vi "SS2 Live_Image Histogram.vi"() -> ()   [LabVIEW 2019]
uses:
  SS2 Live_Settings List.ctl
  Histograms/Linear Histogram Options.ctl
  Histograms/Histogram Bin Position.ctl
  SS2 DAQ Parameters 3.ctl
  SS2 Gate Definition.ctl
  Calc/Conditional Add 1.llb/Conditional Add 1 [I32].vi
  3eb8dcdc-dfa2-4210-84d8-37bed86b0045.vi/f50f8d4e-175f-4c35-82a4-475d9581d4c4.vi
  3eb8dcdc-dfa2-4210-84d8-37bed86b0045.vi/09f68343-6027-4db5-902e-d62cfc368e59.vi
  3eb8dcdc-dfa2-4210-84d8-37bed86b0045.vi/a7808a9a-c229-4fc4-888b-173237c7e755.vi
  3eb8dcdc-dfa2-4210-84d8-37bed86b0045.vi/34d4bd40-5cc8-4a17-aeb0-05577f0cdd25.vi
  3eb8dcdc-dfa2-4210-84d8-37bed86b0045.vi/9e4b3444-9466-44f3-aaf5-79fcd1be1b69.vi
  3eb8dcdc-dfa2-4210-84d8-37bed86b0045.vi/f50f8d4e-175f-4c35-82a4-475d9581d4c4.vi/53a1494f-7830-4d35-b2a0-1dde755757cb.vi
  GUI/Dialog Window with Option.vi
  <vilib>/Analysis/baseanly.llb/Std Deviation and Variance.vi
  <vilib>/Utility/error.llb/Error Cluster From Error Code.vi
  Variant/Variant to Data/Variant to Data.lvlib
panel:
  out "Image Histogram":cluster{"Axis":dbl[], "Histogram":dbl[]}(graph)
  in  "Stop":bool
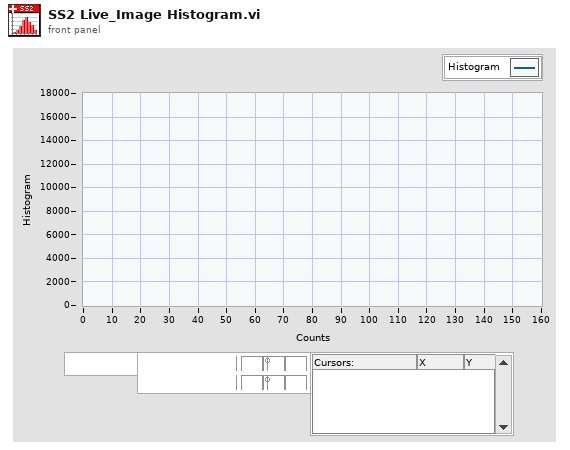
[diagram p1: front panel]
types:
  T1 = typedef "SS2 DAQ Parameters 3.ctl" = cluster{"10 bits":bool, "# Exposure Sequences":u32, "# 1-bit Frame per Gate":u32, "Gate Shift":u32, "# Gates per Set":u32, "# Sets":u32, "Laser Period":dbl[unit], "Sync Period":dbl[unit], "Gate Offset":u32, "Auto-adjust Gate Offset":bool, "Gate Definition":T2}
  T2 = typedef "SS2 Gate Definition.ctl" = cluster{"gs_psincdec_0":u32, "gs_psincdec_1":u32, "gs_psincdec_2":u32, "gs_psincdec_3":u32, "gs_no_shift_adj_1":u32, "gs_no_shift_adj_2":u32, "gs_no_shift_adj_3":u32}
  T3 = typedef "SS2 Live_Settings List.ctl" = enum16{"FPGA:Bitfile Path", "FPGA:Bitfile Version", "FPGA:Auto Reset FPGA", "Acquisition Parameters:SS2 DAQ Parameters", "Acquisition Parameters:Gate Configuration Array", "Acquisition Parameters:Buffer Size (# Gates)", "File Information:File Information", "File Information:# Datasets in Series", "File Information:Scrambled File Flag", "File Information:Delay between Datasets", "Image Parameters:Image ROI Information", "Image Parameters:Image Binning Options", "UI Settings:Histogram Bins Number"}
  T4 = typedef "Linear Histogram Options.ctl" = cluster{"Bin Size":dbl, "Min Value":dbl, "Max Value":dbl, "Filter NaN & Infinite Values":bool, "Frequency Plot":bool, "Align Bins":bool, "Bin Location":T5, "Project Outside Values":bool, "Max Histogram Size":i32}
  T5 = typedef "Histogram Bin Position.ctl" = enum16{"Left", "Center", "Right"}
  T6 = typedef "Array Statistics.ctl" = cluster{"Mean":dbl, "Standard Deviation":dbl, "Max":dbl, "Min":dbl}
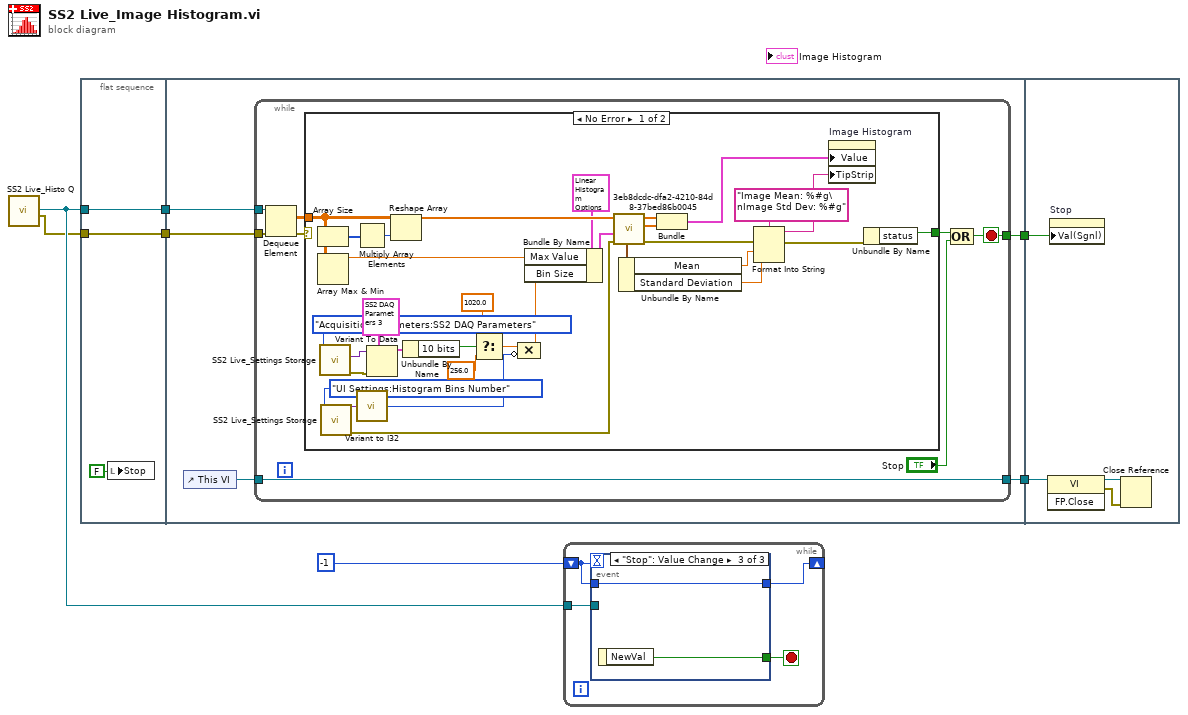
[diagram p0: block diagram]
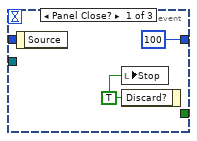
[diagram p2: hidden frame]
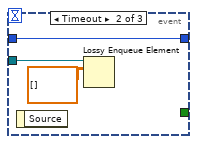
[diagram p3: hidden frame]
diagram:
  n1 = call "SS2 Live_Histo Q.vi"() -> ("error out"=w1:errorcluster, "SS2 Live Histo Q"=w2:refnum<queue>)  [unwired: 6 in]
  n2 = flat-sequence {
    tunnel: [w9] -> w4
    tunnel: w2 -> [w9]
    tunnel: [w8] -> w3
    tunnel: w1 -> [w8]
    tunnel: [w14] -> w7
    tunnel: [w13] -> w6
    tunnel: w4 -> [w12]
    tunnel: w3 -> [w11]
    tunnel: w7 -> [w59]
    tunnel: w6 -> [w58]
    frame #0 {
      n3 = local write "Stop"(FALSE ("Stop")) -> ()
    }
    frame #1 {
      n4 = control-ref of="This VI"() -> (w15:refnum<vi>)
      n5 = while {
        tunnel: w15 -> [w20]
        tunnel: [w20] -> w13
        tunnel: [w18] -> w14
        tunnel: w12 -> [w17]
        tunnel: w11 -> [w16]
        stop <- w18 stop-if-true
        n6 = Dequeue Element(queue=w17, error in (no error)=w16) -> (element=w22:sgl[][], error out=w23:errorcluster)  [unwired: 1 in, 2 out]
        n7 = case shown="No Error" w23 {
          tunnel: w22 -> [w38 _]
          tunnel: [w52 _] -> w21
          frame No Error {
            n8 = Array Size(array=w38) -> (size(s)=w51:i32[])
            n9 = Array Max & Min(array=w38) -> (max value=w36:sgl)  [unwired: 3 out]
            n10 = call "SS2 Live_Settings Storage.vi"("Settings List"=SS2_Live_Settings_List."Acquisition Parameters:SS2 DAQ Parameters") -> ("Error Out"=w33:errorcluster, "Variant Data out"=w32:variant)  [unwired: 9 in]
            n11 = call "SS2 Live_Settings Storage.vi"("Settings List"=SS2_Live_Settings_List."UI Settings:Histogram Bins Number") -> ("Error Out"=w48:errorcluster, "Variant Data out"=w54:variant)  [unwired: 9 in]
            n12 = Multiply Array Elements(1:w51) -> (0:w50:i32)
            n13 = call "Variant to I32.vi"("Variant"=w54) -> ("Value"=w25:i32)  [unwired: 8 in]
            n14 = Variant To Data(error in=w33, type=T1 {"10 bits"=FALSE, "# Exposure Sequences"=0, "# 1-bit Frame per Gate"=255, "Gate Shift"=0, "# Gates per Set"=0, "# Sets"=1, "Laser Period"=0.0, "Sync Period"=0.0, "Gate Offset"=0, "Auto-adjust Gate Offset"=FALSE, "Gate Definition"={"gs_psincdec_0"=0, "gs_psincdec_1"=0, "gs_psincdec_2"=0, "gs_psincdec_3"=0, "gs_no_shift_adj_1"=0, "gs_no_shift_adj_2"=0, "gs_no_shift_adj_3"=0}} ("SS2 DAQ Parameters"), Variant=w32) -> (data=w30:T1)  [unwired: 1 out]
            n15 = Reshape Array(w38, w50) -> (w49:sgl[])
            n16 = Unbundle By Name(w30) -> ("10 bits"=w29:bool)
            n17 = Select(t=1020.0, s=w29, f=256.0) -> (s? t:f=w26:dbl)
            n18 = Compound Arithmetic op=MULTIPLY(w26, invert w25) -> (w24:dbl)
            n19 = Bundle By Name(cluster=T4 {"Bin Size"=nan, "Min Value"=0.0, "Max Value"=inf, "Filter NaN & Infinite Values"=TRUE, "Frequency Plot"=FALSE, "Align Bins"=TRUE, "Bin Location"=enum."Left", "Project Outside Values"=FALSE, "Max Histogram Size"=100000} ("Histogram Options"), "Max Value"=w36, "Bin Size"=w24) -> (w35:T4)
            n20 = call "3eb8dcdc-dfa2-4210-84d8-37bed86b0045.vi"("Error In"=w48, "Histogram Options"=w35, "Array"=w49) -> ("Error Out"=w47:errorcluster, "Array Statistics"=w46:T6, "Histogram"=w42:dbl[], "Axis"=w43:dbl[])  [unwired: 4 in, 1 out]
            n21 = Unbundle By Name(w46) -> ("Mean"=w45:dbl, "Standard Deviation"=w44:dbl)
            n22 = Bundle("Axis"=w43, "Histogram"=w42) -> (w40:cluster{"Axis":dbl[], "Histogram":dbl[]})  [unwired: 1 in]
            n23 = Format Into String(format string="Image Mean: %#g\nImage Std Dev: %#g", error in=w47, w45, w44) -> (resulting string=w39:string, error out=w41:errorcluster)  [unwired: 1 in]
            n24 = property on="Image Histogram" class="XYGraph (strict)"("Value"=w40, "TipStrip"=w39) -> ()  [unwired: 2 in, 2 out]
            n25 = Unbundle By Name(w41) -> ("status"=w52:bool)
          }
          frame Error {
          }
        }
        n26 = Compound Arithmetic op=OR(w21, "Stop") -> (w18:bool)
      }
    }
    frame #2 {
      n27 = invoke class="VI" method="FP.Close"(reference=w58) -> (reference out=w57:refnum<vi>, error out=w56:errorcluster)  [unwired: 2 in, 1 out]
      n28 = property on="Stop" class="Bool (strict)"("Val(Sgnl)"=w59) -> ()  [unwired: 2 in, 2 out]
      n29 = Close Reference(reference=w57, error in (no error)=w56) -> ()  [unwired: 1 out]
    }
  }
  n30 = while {
    tunnel: w2 -> [w62]
    shift-right: [w61] -> _
    shift-left: -1 -> [w60]
    stop <- w63 stop-if-true
    n31 = event shown="[2] \"Stop\": Value Change" {
      selector: _ -> [_ _ _]
      dyn-events: _ -> [_ _ _]
      timeout: w60 -> [_ _ _]
      tunnel: [_ _ w70] -> w63
      tunnel: w62 -> [_ w68 _]
      tunnel: [100 w67 w69] -> w61
      tunnel: w60 -> [_ w67 w69]
      event Panel Close? {
        w64 = TRUE ("Discard?")
        n32 = event-data() -> ()  [unwired: 1 in, 1 out]
        n33 = local write "Stop"(w64) -> ()
        n34 = event-data("Discard?"=w64) -> ()  [unwired: 1 in, 1 out]
      }
      event Timeout {
        n35 = event-data() -> ()  [unwired: 1 in, 1 out]
        n36 = Lossy Enqueue Element(queue=w68, element=sgl[][] []) -> ()  [unwired: 1 in, 4 out]
      }
      event "Stop": Value Change {
        n37 = event-data() -> ("NewVal"=w70:bool)  [unwired: 1 in]
      }
    }
  }
